vi "NodeCount.vi"(8 "error in (no error)":errorcluster, 9 "countedNodes in":refnum<data-value>[](array[refnum]), 10 "count in":u32, 11 "GraphNode in":refnum<class "GraphNode.lvclass">) -> (0 "error out":errorcluster, 1 "countedNodes out":refnum<data-value>[](array[refnum]), 2 "count out":u32, 3 "GraphNode out":refnum<class "GraphNode.lvclass">)   [LabVIEW 2009, in "GraphNode.lvclass"]
uses:
  GraphNode.lvclass
  DataObj/DataObj.lvclass
  Node/Node.lvclass
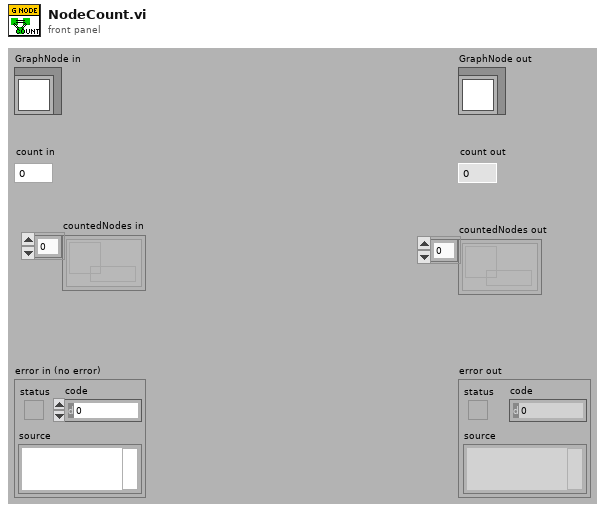
[diagram p1: front panel]
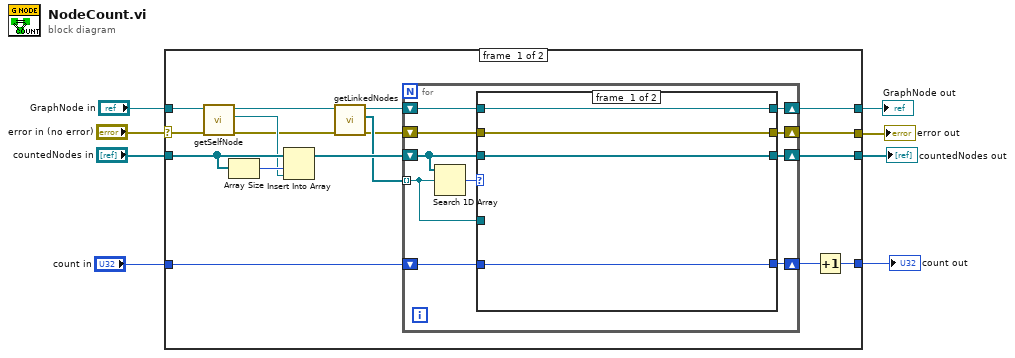
[diagram p0: block diagram]
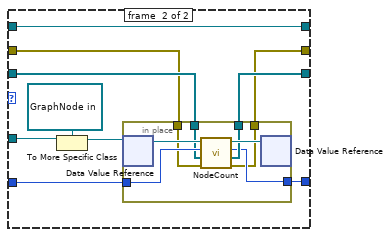
[diagram p2: hidden frame]
diagram:
  n1 = case shown="No Error" "error in (no error)" {
    selector: "error in (no error)" -> [w20 w61]
    tunnel: [w9 w61] -> w7
    tunnel: [w12 w60] -> w6
    tunnel: "GraphNode in" -> [w25 w60]
    tunnel: "count in" -> [w16 w58]
    tunnel: "countedNodes in" -> [w23 w59]
    tunnel: [w13 w59] -> w2
    tunnel: [w10 w58] -> w1
    frame #0 {
      n2 = call "getSelfNode.vi"("error in (no error)"=w20, "Node in"=w25) -> ("error out"=w19:errorcluster, "selfNode"=w22:refnum<data-value>, "Node out"=w21:refnum<class "GraphNode.lvclass">)  [unwired: 7 in]
      n3 = Array Size(array=w23) -> (size(s)=w24:i32)
      n4 = Insert Into Array(array=w23, index=w24, new element=w22) -> (w18:refnum<data-value>[])
      n5 = call "getLinkedNodes.vi"("error in (no error)"=w19, "GraphNode in"=w21) -> ("error out"=w15:errorcluster, "LinkedNodes"=w17:refnum<data-value>[], "GraphNode out"=w14:refnum<class "GraphNode.lvclass">)  [unwired: 7 in]
      n6 = for {
        tunnel: w17 -> [w34] mode=indexing
        shift-right: [w26] -> w9
        shift-left: w15 -> [w27]
        shift-right: [w31] -> w12
        shift-left: w14 -> [w32]
        shift-right: [w29] -> w13
        shift-left: w18 -> [w30]
        shift-right: [w28] -> w11
        shift-left: w16 -> [w33]
        n7 = Search 1D Array(1D array=w30, element=w34) -> (index of element=w35:i32)  [unwired: 1 in]
        n8 = case shown="-1" w35 {
          tunnel: w34 -> [_ w49]
          tunnel: w33 -> [w36 w46]
          tunnel: w32 -> [w39 w45]
          tunnel: [w39 w45] -> w31
          tunnel: w30 -> [w38 w44]
          tunnel: [w38 w43] -> w29
          tunnel: [w36 w42] -> w28
          tunnel: w27 -> [w37 w41]
          tunnel: [w37 w40] -> w26
          frame #0 {
          }
          frame #1 {
            n9 = To More Specific Class(target class=refnum<data-value> refnum ("data value reference"), reference=w49) -> (specific class reference=w47:refnum<data-value>)  [unwired: 1 in, 1 out]
            n10 = in-place {
              in-place-border: w46 -> [w55]
              in-place-border: w44 -> [w54]
              in-place-border: [w53] -> w43
              in-place-border: [w52] -> w42
              in-place-border: w41 -> [w51]
              in-place-border: [w50] -> w40
              n11 = in-place-dvr #1(w47) -> (w57:refnum<class "GraphNode.lvclass">)  [unwired: 1 out]
              n12 = call "NodeCount.vi"("error in (no error)"=w51, "countedNodes in"=w54, "count in"=w55, "GraphNode in"=w57) -> ("error out"=w50:errorcluster, "countedNodes out"=w53:refnum<data-value>[], "count out"=w52:u32, "GraphNode out"=w56:refnum<class "GraphNode.lvclass">)  [unwired: 4 in]
              n13 = in-place-dvr #1(w56) -> ()  [unwired: 2 out]
            }
          }
        }
      }
      n14 = Increment(x=w11) -> (x+1=w10:u32)
    }
    frame #1 {
    }
  }
  "error out" <- w7
  "GraphNode out" <- w6
  "count out" <- w1
  "countedNodes out" <- w2
